vi "Write Stop Bits.vi"(8 "error in (no error)":errorcluster caption="错误输入（无错误）", 10 "Stop Bits":u16(ring)=10 items=["1.0"=10, "1.5"=15, "2.0"=20], 11 "Serial Slave输入":refnum<class "Serial Slave.lvclass">) -> (0 "error out":errorcluster caption="错误输出", 3 "Serial Slave输出":refnum<class "Serial Slave.lvclass">)   [LabVIEW 2013, in "Modbus Library - Advance.lvlib" / "Serial Slave.lvclass"]
uses:
  Serial Slave.lvclass
  Serial Slave.lvclass/Serial Slave.ctl
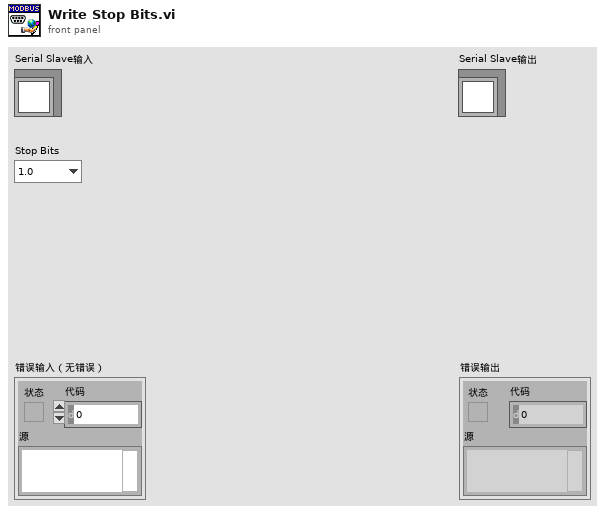
[diagram p1: front panel]
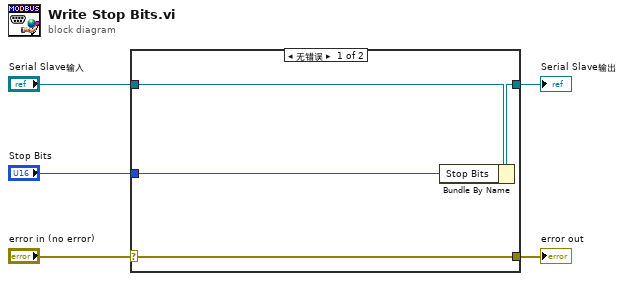
[diagram p0: block diagram]
diagram:
  n1 = case shown="无错误" "error in (no error)" {
    selector: "error in (no error)" -> [w9 w10]
    tunnel: [w9 w10] -> w4
    tunnel: [w7 w11] -> w2
    tunnel: "Serial Slave输入" -> [w8 w11]
    tunnel: "Stop Bits" -> [w6 _]
    frame No Error {
      n2 = Bundle By Name(cluster=w8, "Stop Bits"=w6) -> (w7:refnum<class "Serial Slave.lvclass">)
    }
    frame Error {
    }
  }
  "error out" <- w4
  "Serial Slave输出" <- w2
